vi "Append to display log.vi"(8 "error in":errorcluster, 9 "Num Entries":i32=40, 11 "string":string) -> (0 "error out":errorcluster)   [LabVIEW 2018]
uses:
  CAEN globals.vi
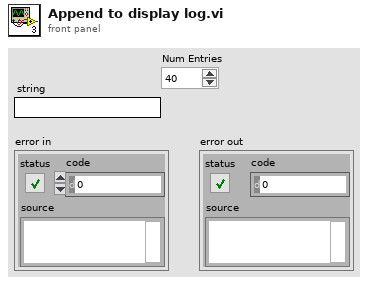
[diagram p1: front panel]
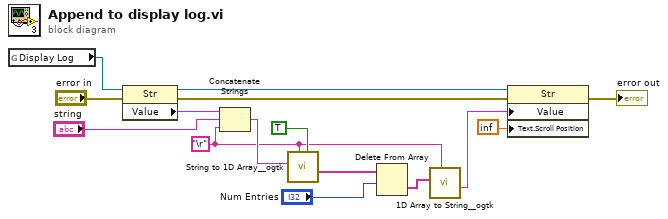
[diagram p0: block diagram]
diagram:
  w4 = "\r"
  n1 = global read "CAEN globals.vi" "Display Log"() -> (w9:refnum<vi>)
  n2 = property class="Str"(reference=w9, error in="error in") -> (reference out=w11:refnum<vi>, error out=w12:errorcluster, "Value"=w10:string)
  n3 = Concatenate Strings(w10, "string", w4) -> (w8:string)
  n4 = call <userlib>:"String to 1D Array__ogtk.vi"("ignore duplicate delimiters? (F=No)"=TRUE, "delimiter (Tab)"=w4, "string"=w8) -> ("Array of Strings"=w6:string[])  [unwired: 8 in]
  n5 = Delete From Array(array=w6, length="Num Entries") -> (deleted portion=w5:string[])  [unwired: 1 in, 1 out]
  n6 = call <userlib>:"1D Array to String__ogtk.vi"("delimiter (Tab)"=w4, "Array of Strings"=w5) -> ("delimited string"=w3:string)  [unwired: 9 in]
  n7 = property class="Str"(reference=w11, error in=w12, "Value"=w3, "Text.Scroll Position"=inf) -> (error out=→"error out":errorcluster)  [unwired: 1 out]
